vi "Run 01.vi"   [LabVIEW 2016]
types:
  T1 = typedef "LVHSConnector.ctl" = refnum<class "BrickReference.lvclass">
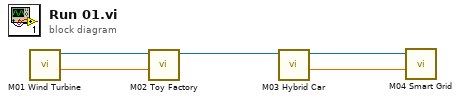
[diagram p0: block diagram]
diagram:
  n1 = call "M01 Wind Turbine.vi"() -> ("Angle out"=w4:sgl, "EV3 out"=w5:T1)  [unwired: 10 in]
  n2 = call "M02 Toy Factory.vi"("Angle in"=w4, "EV3 in"=w5) -> ("EV3 out"=w3:T1)  [unwired: 9 in]
  n3 = call "M03 Hybrid Car.vi"("EV3 in"=w3) -> ("Angle out"=w1:sgl, "EV3 out"=w2:T1)  [unwired: 9 in]
  n4 = call "M04 Smart Grid.vi"("Target angle"=w1, "EV3 in"=w2) -> ()  [unwired: 9 in, 1 out]
